vi "create.vi"(8 "error in (no error)":errorcluster, 11 "IOvenFactory":refnum<class "IOvenFactory.lvclass">) -> (0 "error out":errorcluster, 3 "OvenController out":refnum<class "OvenController.lvclass">)   [LabVIEW 2023, in "AbstractFactory.lvlib" / "OvenController.lvclass"]
uses:
  OvenController.lvclass
  IOvenFactory/IOvenFactory.lvclass
  OvenController.lvclass/OvenController.ctl
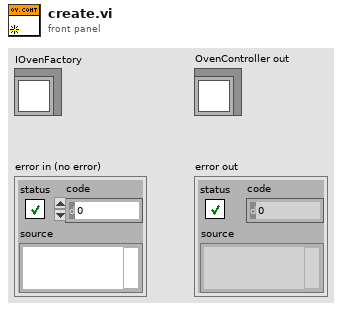
[diagram p1: front panel]
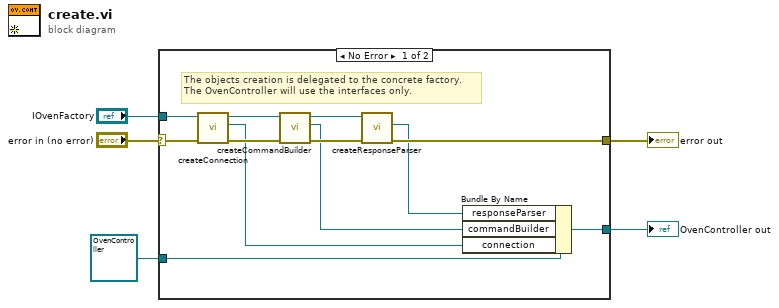
[diagram p0: block diagram]
diagram:
  n1 = case shown="No Error" "error in (no error)" {
    selector: "error in (no error)" -> [w14 w19]
    tunnel: [w13 w19] -> w4
    tunnel: [w9 w18] -> w2
    tunnel: refnum<class "OvenController.lvclass"> refnum ("OvenController in") -> [w17 w18]
    tunnel: "IOvenFactory" -> [w12 _]
    frame No Error {
      # "The objects creation is delegated to the concrete factory.\nThe OvenController will use the interfaces only."
      n2 = call-dynamic "createConnection.vi"("error in (no error)"=w14, "IOvenFactory in"=w12) -> ("error out"=w16:errorcluster, "connection"=w6:refnum<class "IConnection.lvclass">, "IOvenFactory out"=w11:refnum<class "IOvenFactory.lvclass">)  [unwired: 7 in]
      n3 = call-dynamic "createCommandBuilder.vi"("error in (no error)"=w16, "IOvenFactory in"=w11) -> ("error out"=w15:errorcluster, "commandBuilder"=w7:refnum<class "ICommandBuilder.lvclass">, "IOvenFactory out"=w10:refnum<class "IOvenFactory.lvclass">)  [unwired: 7 in]
      n4 = call-dynamic "createResponseParser.vi"("error in (no error)"=w15, "IOvenFactory in"=w10) -> ("error out"=w13:errorcluster, "responseParser"=w8:refnum<class "IResponseParser.lvclass">)  [unwired: 7 in, 1 out]
      n5 = Bundle By Name(cluster=w17, "responseParser"=w8, "commandBuilder"=w7, "connection"=w6) -> (w9:refnum<class "OvenController.lvclass">)
    }
    frame Error {
    }
  }
  "error out" <- w4
  "OvenController out" <- w2
